vi "SCMP - FW init.vi"(7 "FW refs":refnum<vi>[](array[refnum]), 8 "error in (no error)":errorcluster, 11 "FITS Header in":T1={"Wavelength (nm)"=530.15, "Exposure (s)"=0.05, "Tuning Delay (ms)"=200.0, "Beam Type (-1/1)"=1.0, "Tuning Voltages"=[1.111, 2.222, 3.333, 4.444], "Observer"="observer", "Light Shapping Diffuser"=enum."In Beam", "Comment"="", "Data Type"=enum."LIVE", "Mod Cycles"=1, "SCD Calibration Optics"=enum."1 - Polarizer @0, I+Q", "SCD Emission Line Filter"=enum."1-557.6nm", "Cookbook"="", "COMP-S Calibration Wheel"=enum."Dark", "COMP-S Andover Filter Wheel"=enum."530.3nm/HWB 0.34nm (Fe XIV)", "FOV Rotation (deg)"=66.0, "Objective Lens Position (mm)"=0.0, "Occulter size"=0.0, "Time End"=timestamp(3382374145.421875 s since 1904-01-01), "Acc Exposure (s)"=0.0, "Time Stamp Array"=[], "Camera Serial Number"=[], "Camera Temp"=[], "Camera PI (mm)"=[0.0, 0.0, 0.0], "Time Start"=timestamp(3382374145.421875 s since 1904-01-01), "Peripherals"={"ILX controler"=FALSE, "Zone temperatures"=FALSE, "Andor"=FALSE, "Andor 2"=FALSE, "PI Stages"=FALSE, "AISAS mechanisms"=FALSE, "AISAS Mech.lvclass"=refnum, "Zone temp ref"=variant, "FWs"=FALSE}, "FITS paths"=[], "Cameras"=enum."Andor", "load preset cbk"=FALSE, "periodic check count"=0, "COMP-S Calibration Wheel 2"=enum."Dark", "Calib"=enum."Dark", "Abso Aperture"=66.0, "Nominal Aperture"=66.0, "Pointer IP"="127.0.0.1"} {"Nominal Aperture" format="%.1f"; "Abso Aperture" format="%.1f"; "Camera PI (mm)" format="%_3g"; "Acc Exposure (s)" format="%^.3g"; "Occulter size" format="%.2f"; "Objective Lens Position (mm)" min=70.0 max=152.0 format="%.2f"; "FOV Rotation (deg)" format="%.1f"; "Exposure (s)" format="%^.3g"; "Wavelength (nm)" format="%_6g"}) -> (0 "error out":errorcluster, 3 "FITS Header out":T1={"Wavelength (nm)"=0.0, "Exposure (s)"=0.0, "Tuning Delay (ms)"=0.0, "Beam Type (-1/1)"=0.0, "Tuning Voltages"=[], "Observer"="", "Light Shapping Diffuser"=enum."Out of Beam", "Comment"="", "Data Type"=enum."LIVE", "Mod Cycles"=0, "SCD Calibration Optics"=enum."1 - Polarizer @0, I+Q", "SCD Emission Line Filter"=enum."1-557.6nm", "Cookbook"="", "COMP-S Calibration Wheel"=enum."Dark", "COMP-S Andover Filter Wheel"=enum."530.3nm/HWB 0.34nm (Fe XIV)", "FOV Rotation (deg)"=0.0, "Objective Lens Position (mm)"=0.0, "Occulter size"=0.0, "Time End"=timestamp(0 s since 1904-01-01), "Acc Exposure (s)"=0.0, "Time Stamp Array"=[], "Camera Serial Number"=[], "Camera Temp"=[], "Camera PI (mm)"=[], "Time Start"=timestamp(0 s since 1904-01-01), "Peripherals"={"ILX controler"=FALSE, "Zone temperatures"=FALSE, "Andor"=FALSE, "Andor 2"=FALSE, "PI Stages"=FALSE, "AISAS mechanisms"=FALSE, "AISAS Mech.lvclass"=refnum, "Zone temp ref"=variant, "FWs"=FALSE}, "FITS paths"=[], "Cameras"=enum."Andor", "load preset cbk"=FALSE, "periodic check count"=0, "COMP-S Calibration Wheel 2"=enum."Dark", "Calib"=enum."Dark", "Abso Aperture"=66.0, "Nominal Aperture"=66.0, "Pointer IP"="127.0.0.1"} {"Nominal Aperture" format="%.1f"; "Abso Aperture" format="%.1f"; "Camera PI (mm)" format="%_3g"; "Acc Exposure (s)" format="%^.3g"; "Occulter size" format="%.2f"; "Objective Lens Position (mm)" min=70.0 max=152.0 format="%.2f"; "FOV Rotation (deg)" format="%.1f"; "Exposure (s)" format="%^.3g"; "Wavelength (nm)" format="%_6g"})   [LabVIEW 2014]
uses:
  Controls/SCD - FITS Cluster.ctl
  AISAS/Mech/AISAS Mech.lvclass
  AISAS/Controls/Diffuser.ctl
  Controls/FITS Data type.ctl
  Controls/SCD - Calibration Optics Filter Wheel.ctl
  Controls/SCD - EDT - Emission Line Filter Wheel.ctl
  Controls/CoMP-S Controls/Polarization Optics Filter Wheel.ctl
  Controls/CoMP-S Controls/Emission Line Filter Wheel.ctl
  AISAS/Controls/focus.ctl
  Controls/peripherals.ctl
  Controls/Cameras select.ctl
  Controls/Globals.vi
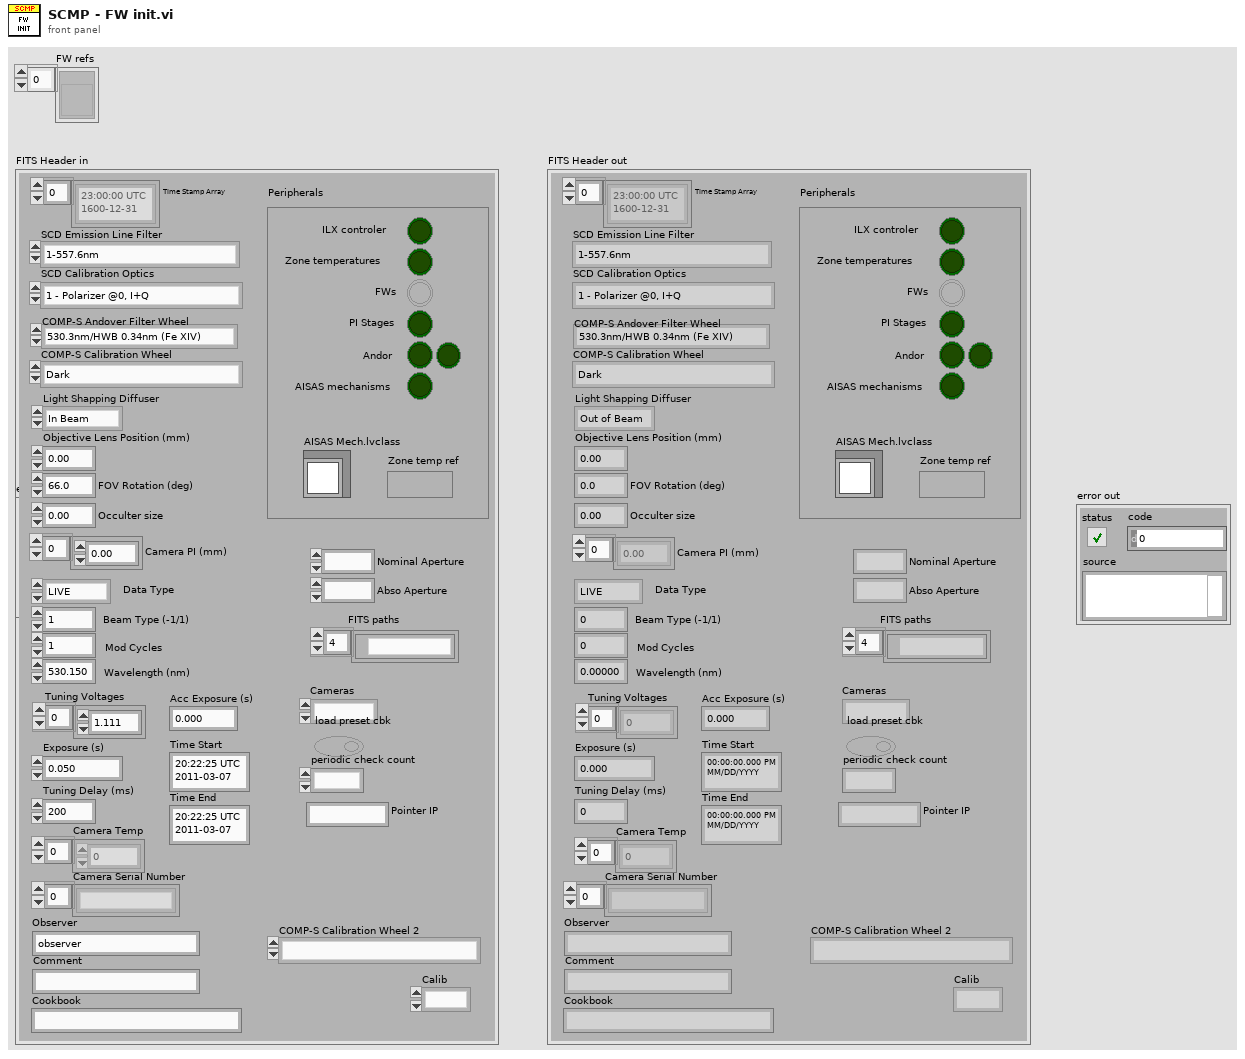
[diagram p1: front panel]
types:
  T1 = typedef "SCD - FITS Cluster.ctl" = cluster{"Wavelength (nm)":dbl, "Exposure (s)":dbl, "Tuning Delay (ms)":dbl, "Beam Type (-1/1)":dbl, "Tuning Voltages":dbl[], "Observer":string, "Light Shapping Diffuser":T2, "Comment":string, "Data Type":T3, "Mod Cycles":u16, "SCD Calibration Optics":T4, "SCD Emission Line Filter":T5, "Cookbook":string, "COMP-S Calibration Wheel":T6, "COMP-S Andover Filter Wheel":T7, "FOV Rotation (deg)":dbl, "Objective Lens Position (mm)":T8, "Occulter size":dbl, "Time End":timestamp, "Acc Exposure (s)":dbl, "Time Stamp Array":timestamp[], "Camera Serial Number":string[], "Camera Temp":dbl[], "Camera PI (mm)":dbl[], "Time Start":timestamp, "Peripherals":T9, "FITS paths":path[], "Cameras":T10, "load preset cbk":bool, "periodic check count":i32, "COMP-S Calibration Wheel 2":T6, "Calib":enum16{"Dark", "Flat"}, "Abso Aperture":dbl, "Nominal Aperture":dbl, "Pointer IP":string}
  T2 = typedef "Diffuser.ctl" = enum16{"Out of Beam", "In Beam"}
  T3 = typedef "FITS Data type.ctl" = enum16{"LIVE", "DARK", "FLAT", "CALI", "OBSE", "ABSO", "AURE", "TARG", "OBJE", "HOLE", "OREX", "THRO", "CHIP"}
  T4 = typedef "SCD - Calibration Optics Filter Wheel.ctl" = enum16{"1 - Polarizer @0, I+Q", "2 - Polarizer @90, I-Q", "3 - Polarizer @45, I+U", "4 - Polarizer @135, I-U", "5 - Polarizer @0, Retarder @45, I+V", "6 - Polarizer @0, Retarder @135, I-V", "7 - Dark", "8 - Clear", "9 - N/A"}
  T5 = typedef "SCD - EDT - Emission Line Filter Wheel.ctl" = enum16{"1-557.6nm", "2-587.6nm", "3-589.6nm", "4-630.2nm", "5-656.4nm", "6-849.8nm", "7-854.2nm", "8-866.2nm", "9-1083.0nm"}
  T6 = typedef "Polarization Optics Filter Wheel.ctl" = enum16{"Dark", "Clear", "Exchange Lens", "Polarizer @0, I+Q", "Polarizer @90, I-Q", "Polarizer @45, I+U", "Polarizer @135, I-U", "Polarizer @0, Retarder @45, I+V", "Polarizer @0, Retarder @135, I-V"}
  T7 = typedef "Emission Line Filter Wheel.ctl" = enum16{"530.3nm/HWB 0.34nm (Fe XIV)", "587.6nm/HBW 0.44nm (He I D3)", "637.5nm/HBW 0.53nm (Fe X)", "656.3nm/HBW 0.57nm (H-Alpha)", "789.2nm/HBW 0.85nm (Fe XI)", "854.2nm/HBW 1.01nm (Ca I)", "1074.7nm/HBW 2.34nm (Fe XIII)", "1079.8nm/HBW 1.64nm (Fe XIII)", "1083.0nm/HBW 1.66nm (He I)"}
  T8 = typedef "focus.ctl" = dbl
  T9 = typedef "peripherals.ctl" = cluster{"ILX controler":bool, "Zone temperatures":bool, "Andor":bool, "Andor 2":bool, "PI Stages":bool, "AISAS mechanisms":bool, "AISAS Mech.lvclass":refnum<class "AISAS Mech.lvclass">, "Zone temp ref":variant, "FWs":bool}
  T10 = typedef "Cameras select.ctl" = enum16{"Andor", "GDR"}
  T11 = enum16{"Emission Line Filters", "Calibration Polarizers"}
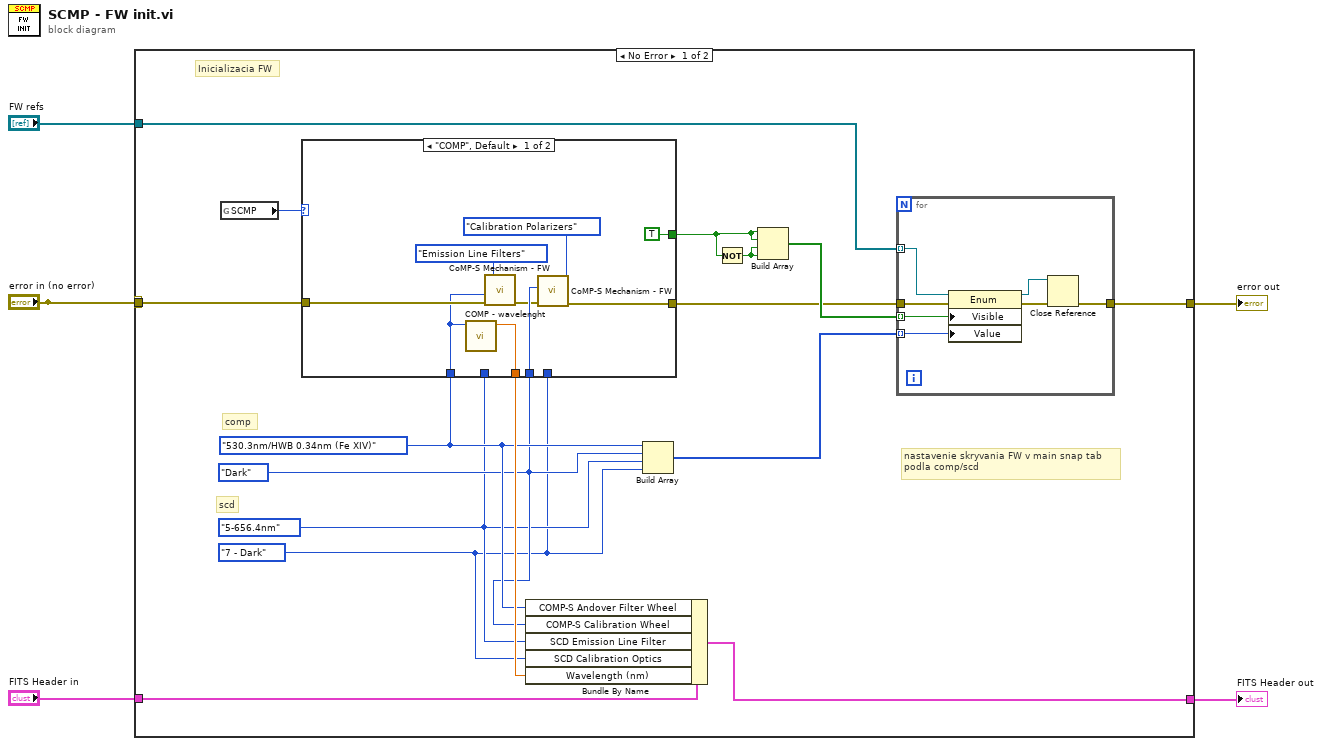
[diagram p0: block diagram]
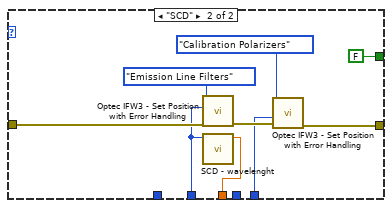
[diagram p2: hidden frame]
diagram:
  n1 = case shown="No Error" "error in (no error)" {
    selector: "error in (no error)" -> [_ w48]
    tunnel: "error in (no error)" -> [w20 _]
    tunnel: [w9 w47] -> w5
    tunnel: "FITS Header in" -> [w19 w47]
    tunnel: [w7 w48] -> w3
    tunnel: "FW refs" -> [w6 _]
    frame No Error {
      w12 = SCD_-_EDT_-_Emission_Line_Filter_Wheel."5-656.4nm" ("SCD Emission Line Filter")
      w11 = SCD_-_Calibration_Optics_Filter_Wheel."7 - Dark" ("Calibration Optics")
      w17 = Polarization_Optics_Filter_Wheel."Dark" ("Calibration Wheel")
      w18 = Emission_Line_Filter_Wheel."530.3nm/HWB 0.34nm (Fe XIV)" ("Andover Filter Wheel")
      # "Inicializacia FW"
      # "nastavenie skryvania FW v main snap tab\npodla comp/scd"
      # "scd"
      # "comp"
      n2 = global read "Globals.vi" "SCMP"() -> (w13:enum16{"COMP", "SCD"})
      n3 = case shown="\"COMP\", Default" w13 {
        tunnel: [w30 w33] -> w21
        tunnel: w20 -> [w29 w36]
        tunnel: w18 -> [w28 _]
        tunnel: w17 -> [w27 _]
        tunnel: [w26 w35] -> w8
        tunnel: w12 -> [_ w34]
        tunnel: w11 -> [_ w32]
        tunnel: [TRUE ("Visible") FALSE ("Visible")] -> w10
        frame "COMP", Default {
          n4 = call "COMP - wavelenght.vi"("COMP-S Andover Filter Wheel"=w28) -> ("Wavelength (nm)"=w30:dbl)  [unwired: 10 in]
          n5 = call "CoMP-S Mechanism - FW.vi"("error in (no error)"=w29, "Emission Line Filters [530.3 nm]"=w28, "Filter Wheel Selector"=T11."Emission Line Filters") -> ("error out"=w24:errorcluster)  [unwired: 5 in, 3 out]
          n6 = call "CoMP-S Mechanism - FW.vi"("error in (no error)"=w24, "Calibration Polarizer Filters [Dark]"=w27, "Filter Wheel Selector"=T11."Calibration Polarizers") -> ("error out"=w26:errorcluster)  [unwired: 5 in, 3 out]
        }
        frame "SCD" {
          n7 = call "Optec IFW3 - Set Position with Error Handling.vi"("error in"=w36, "Emission Line Filter"=w34, "Filter Wheel Selector"=T11."Emission Line Filters") -> ("error out"=w39:errorcluster)  [unwired: 6 in, 2 out]
          n8 = call "SCD - wavelenght.vi"("SCD Emission Line Filter"=w34) -> ("Numeric"=w33:dbl)  [unwired: 10 in]
          n9 = call "Optec IFW3 - Set Position with Error Handling.vi"("error in"=w39, "SCD Calibration Optics"=w32, "Filter Wheel Selector"=T11."Calibration Polarizers") -> ("error out"=w35:errorcluster)  [unwired: 6 in, 2 out]
        }
      }
      n10 = Bundle By Name(cluster=w19, "COMP-S Andover Filter Wheel"=w18, "COMP-S Calibration Wheel"=w17, "SCD Emission Line Filter"=w12, "SCD Calibration Optics"=w11, "Wavelength (nm)"=w21) -> (w9:T1)
      n11 = Build Array(w18, w17, w12, w11) -> (w16:u16[])
      n12 = Not(x=w10) -> (.not. x?=w15:bool)
      n13 = Build Array(w10, w10, w15, w15) -> (w14:bool[])
      n14 = for {
        tunnel: w16 -> [w45] mode=indexing
        tunnel: w14 -> [w46] mode=indexing
        tunnel: w6 -> [w43] mode=indexing
        tunnel: w8 -> [w44]
        tunnel: [w41] -> w7
        n15 = property class="Enum"(reference=w43, error in=w44, "Visible"=w46, "Value"=w45) -> (reference out=w40:refnum<vi>, error out=w42:errorcluster)
        n16 = Close Reference(reference=w40, error in (no error)=w42) -> (error out=w41:errorcluster)
      }
    }
    frame Error {
    }
  }
  "FITS Header out" <- w5
  "error out" <- w3
